vi "7thOrderExpandedWLC.vi"(0 "Y":dbl[](array[numeric]), 1 "X":dbl[](array[numeric]), 2 "Coefficients":dbl[](array[numeric])) -> (3 "Y converted":dbl[](array[numeric]), 4 "X converted":dbl[](array[numeric]), 5 "Residue":dbl[](array[numeric]), 6 "f(X,a)":dbl[](array[numeric]))   [LabVIEW 2020, in "XYcenter.lvlib"]
uses:
  XYcenter.lvlib
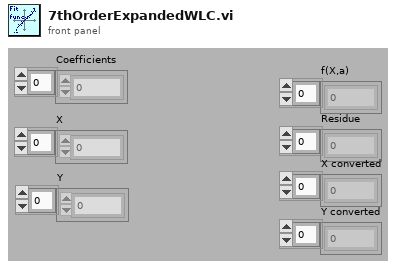
[diagram p1: front panel]
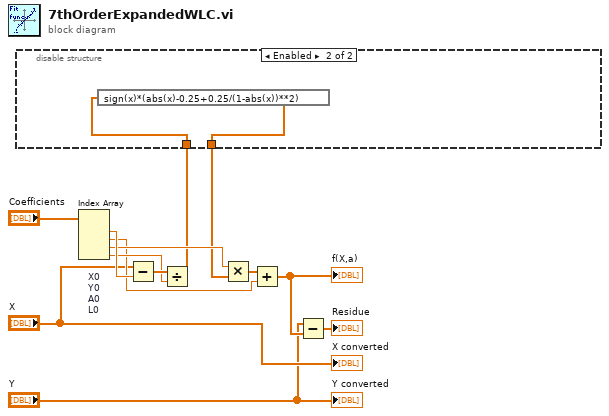
[diagram p0: block diagram]
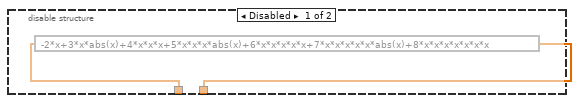
[diagram p2: hidden frame]
diagram:
  n1 = Index Array "X0\nY0\nA0\nL0"(array="Coefficients") -> (element #1=w13:dbl, element #2=w7:dbl, element #3=w12:dbl, element #4=w10:dbl)  [unwired: 4 in]
  n2 = Subtract(x="X", y=w13) -> (x-y=w11:dbl[])
  n3 = Divide(x=w11, y=w10) -> (x/y=w3:dbl[])
  n4 = disable-structure shown="Enabled" {
    disable-tunnel: w3 -> [w15 w17]
    disable-tunnel: [w14 w16] -> w2
    frame Disabled {
      n5 = expression code="-2*x+3*x*abs(x)+4*x*x*x+5*x*x*x*abs(x)+6*x*x*x*x*x+7*x*x*x*x*x*abs(x)+8*x*x*x*x*x*x*x"(w15) -> (w14:dbl[])
    }
    frame Enabled {
      n6 = expression code="sign(x)*(abs(x)-0.25+0.25/(1-abs(x))**2)"(w17) -> (w16:dbl[])
    }
  }
  n7 = Multiply(x=w12, y=w2) -> (x*y=w9:dbl[])
  n8 = Add(x=w9, y=w7) -> (x+y=w4:dbl[])
  "f(X,a)" <- w4
  n9 = Subtract(x="Y", y=w4) -> (x-y=→"Residue":dbl[])
  "X converted" <- "X"
  "Y converted" <- "Y"
